vi "WaitInstanciation.vi"(8 "error in (no error)":errorcluster, 9 "Timeout additional message (\"\")":string, 10 "Timeout [ms]":i32, 11 "Instanciation Notifier":refnum<notifier>) -> (0 "error out":errorcluster, 3 "GLF Instance":refnum<class "IAmGLF.lvclass">)   [LabVIEW 2020, in "GLF.lvlib" / "IAmGLF.lvclass"]
uses:
  IAmGLF.lvclass
  InstanciationNotifierData--cluster.ctl
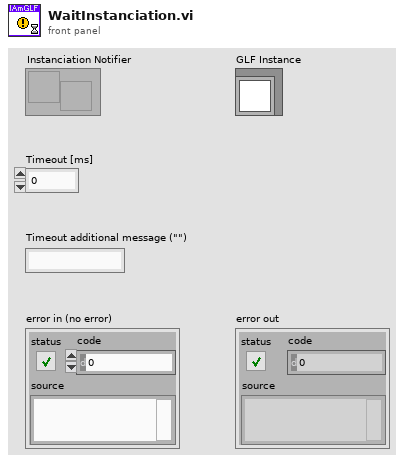
[diagram p1: front panel]
types:
  T1 = typedef "GLF.lvlib/IAmGLF.lvclass/InstanciationNotifierData--cluster.ctl" = cluster{"GLF Instance":refnum<class "IAmGLF.lvclass">, "Error":errorcluster}
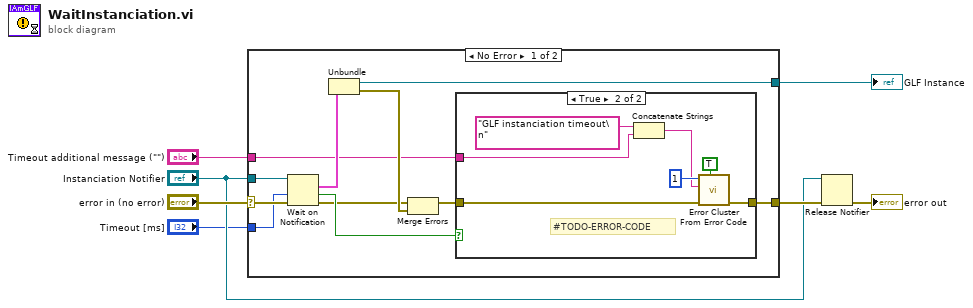
[diagram p0: block diagram]
diagram:
  n1 = case shown="No Error" "error in (no error)" {
    selector: "error in (no error)" -> [w14 w27]
    tunnel: [w13 w27] -> w5
    tunnel: [w12 _] -> w6
    tunnel: "Instanciation Notifier" -> [w11 _]
    tunnel: "Timeout [ms]" -> [w9 _]
    tunnel: "Timeout additional message (\"\")" -> [w8 _]
    frame No Error {
      n2 = Wait on Notification(notifier=w11, timeout in ms (-1)=w9, error in (no error)=w14) -> (notification=w18:T1, timed out?=w15:bool, error out=w10:errorcluster)  [unwired: 1 in, 1 out]
      n3 = Unbundle(w18) -> ("GLF Instance"=w12:refnum<class "IAmGLF.lvclass">, "Error"=w16:errorcluster)
      n4 = Merge Errors(w10, w16) -> (w17:errorcluster)
      n5 = case shown="True" w15 {
        tunnel: w17 -> [w19 w26]
        tunnel: [w19 w25] -> w13
        tunnel: w8 -> [_ w20]
        frame False {
        }
        frame True {
          # "#TODO-ERROR-CODE"
          n6 = Concatenate Strings("GLF instanciation timeout\n" ("error message (\"\")"), w20) -> (w21:string)
          n7 = call <vilib>:"Error Cluster From Error Code.vi"("show call chain? (False)"=TRUE, "error in (no error)"=w26, "error message (\"\")"=w21, "error code (0)"=1) -> ("error out"=w25:errorcluster)  [unwired: 5 in]
        }
      }
    }
    frame Error {
    }
  }
  "GLF Instance" <- w6
  n8 = Release Notifier(notifier="Instanciation Notifier", error in (no error)=w5) -> (error out=→"error out":errorcluster)  [unwired: 1 in, 2 out]
